vi "CALC_PAR_DEL_ALL.vi"(0 "VISA IN":refnum<visa-resource-name>, 5 "error in":errorcluster) -> (14 "VISA Out":refnum<visa-resource-name>, 19 "error out":errorcluster)   [LabVIEW 2018, in "PNA-X.lvlib"]
doc: "CALCulate<cnum>:PARameter:DELete[:NAME] <Mname> \n(Write-only) Deletes the specified measurement. \nSee Critical Note \nParameters \n<cnum> Channel number of the measurement. There must be a selected measurement \non that channel. If unspecified, <cnum> is set to 1. \n<Mname> String - Name of the measurement \nExamples CALC:PAR:DEL 'TEST' \ncalculate2:parameter:delete 'test' \nQuery Syntax Not Applicable \nDefault Not Applicable \nCALCulate:PARameter:DELete:ALL \n1557\n\n(Write-only) Deletes all measurements on the PNA. \nSee Critical Note \nParameters \nExamples CALC:PAR:DEL:ALL \nQuery Syntax Not Applicable \nDefault Not Applicable"
uses:
  PNA-X.lvlib
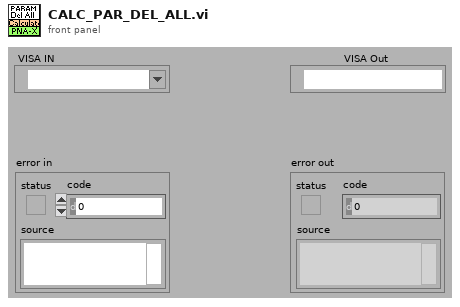
[diagram p1: front panel]
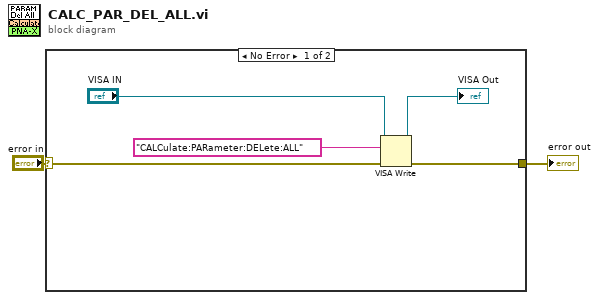
[diagram p0: block diagram]
diagram:
  n1 = case shown="No Error" "error in" {
    selector: "error in" -> [w3 w8]
    tunnel: [w6 w8] -> w1
    frame No Error {
      n2 = VISA Write(VISA resource name="VISA IN", write buffer="CALCulate:PARameter:DELete:ALL" ("Cmdline"), error in (no error)=w3) -> (VISA resource name out=→"VISA Out":refnum<visa-resource-name>, error out=w6:errorcluster)  [unwired: 1 out]
    }
    frame Error {
    }
  }
  "error out" <- w1
